vi "Magnet update rewiring.vi"(6 "output cluster":T1, 9 "Time":timestamp, 10 "Magnet in":T8, 11 "Magnet controls in":T7 {"Output\n[T]" scale=0.0..16.0; "Field\n[T]" scale=0.0..16.0; "Desired ramp\nrate [mT/s]" max=7.545; "Set Field [T]" min=0.0 max=16.0}) -> (2 "Magnet out":T8, 3 "Magnet controls out":T7 {"Output\n[T]" scale=0.0..16.0; "Field\n[T]" scale=0.0..16.0; "Desired ramp\nrate [mT/s]" max=7.545; "Set Field [T]" min=0.0 max=16.0})   [LabVIEW 2024]
uses:
  Subsystem modules/Magnet module/ctl/RampingOutput.ctl
  Datatypes/Magnet controls.ctl
  Subsystem modules/Magnet module/ctl/Overall status.ctl
  Subsystem modules/Magnet module/ctl/SetField data.ctl
  Subsystem modules/Magnet module/ctl/Magnet mode public.ctl
  Subsystem modules/Magnet module/ctl/Actual magnet state.ctl
  Subsystem modules/Magnet module/ctl/Magnet mode.ctl
  Subsystem modules/Magnet module/Magnet module.lvlib
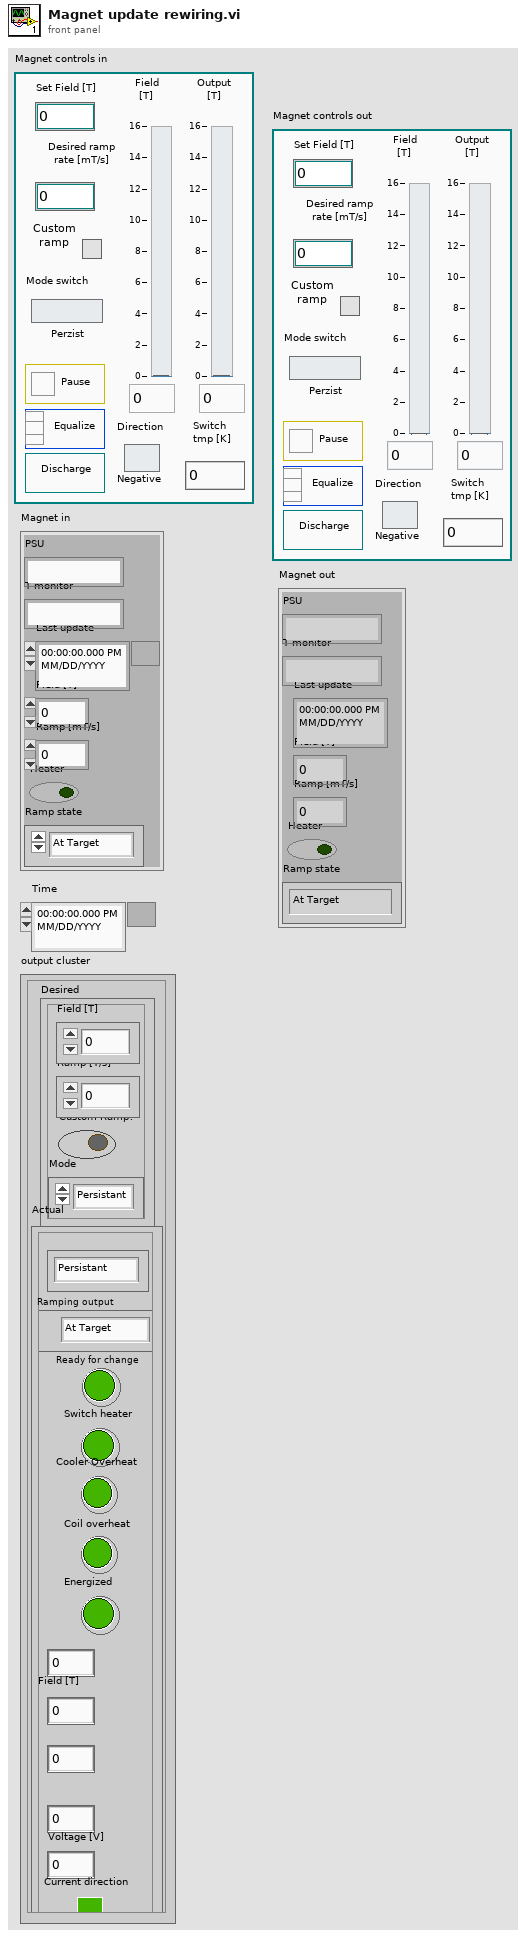
[diagram p1: front panel]
types:
  T1 = typedef "Magnet module.lvlib/Overall status.ctl" = cluster{"Desired":T2, "Actual":T4}
  T2 = typedef "Magnet module.lvlib/SetField data.ctl" = cluster{"Field [T]":dbl, "Ramp [T/s]":dbl, "Custom Ramp?":bool, "Mode":T3}
  T3 = typedef "Magnet module.lvlib/Magnet mode public.ctl" = enum16{"Persistant", "Ramping"}
  T4 = typedef "Magnet module.lvlib/Actual magnet state.ctl" = cluster{"Mode":T5, "Ramping output":T6, "Ready for change":bool, "Switch heater":bool, "Cooler Overheat":bool, "Coil overheat":bool, "Energized":bool, "Output [T]":dbl, "Field [T]":dbl, "Ramp[T/s]":dbl, "Switch\ntemperature [K]":dbl, "Voltage [V]":dbl, "Current direction":bool}
  T5 = typedef "Magnet module.lvlib/Magnet mode.ctl" = enum16{"Persistant", "Switching", "Ramping", "Quenched"}
  T6 = typedef "Magnet module.lvlib/RampingOutput.ctl" = enum16{"At Target", "Go up", "Go down"}
  T7 = typedef "Magnet controls.ctl" = cluster{"Set Field [T]":dbl, "Desired ramp\nrate [mT/s]":dbl, "Custom\nramp":bool, "Mode switch":bool, "Pause ramp":bool, "Field\n[T]":dbl, "Output\n[T]":dbl, "Equalize":bool, "Discharge":bool, "Switch \ntmp [K]":dbl, "Direction":bool}
  T8 = cluster{"PSU":string, "T monitor":string, "Last update":timestamp, "Field [T]":dbl, "Ramp [mT/s]":dbl, "Heater":bool, "Ramp state":T6}
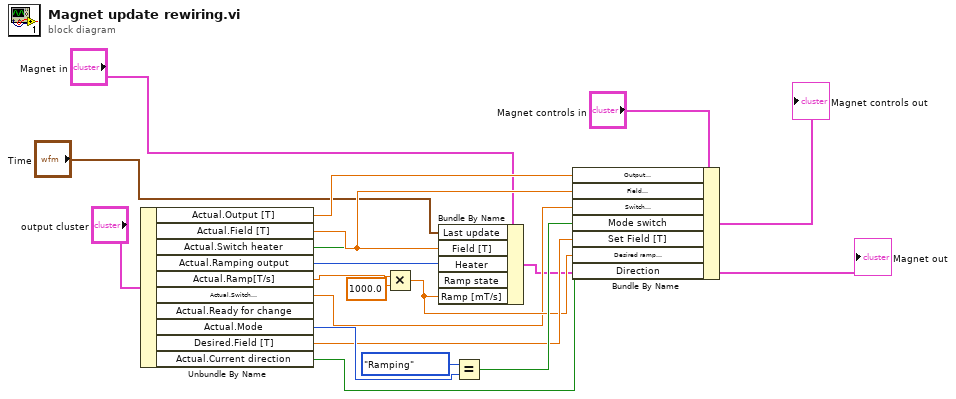
[diagram p0: block diagram]
diagram:
  n1 = Unbundle By Name("output cluster") -> ("Actual.Output [T]"=w10:dbl, "Actual.Field [T]"=w15:dbl, "Actual.Switch heater"=w3:bool, "Actual.Ramping output"=w13:T6, "Actual.Ramp[T/s]"=w11:dbl, "Actual.Switch\ntemperature [K]"=w12:dbl, "Actual.Mode"=w17:T5, "Desired.Field [T]"=w16:dbl, "Actual.Current direction"=w1:bool)  [unwired: 1 out]
  n2 = Multiply(x=w11, y=1000.0) -> (x*y=w14:dbl)
  n3 = Bundle By Name(cluster="Magnet in", "Last update"="Time", "Field [T]"=w15, "Heater"=w3, "Ramp state"=w13, "Ramp [mT/s]"=w14) -> (→"Magnet out":T8)
  n4 = Equal?(x=Magnet_mode."Ramping", y=w17) -> (x = y?=w19:bool)
  n5 = Bundle By Name(cluster="Magnet controls in", "Output\n[T]"=w10, "Field\n[T]"=w15, "Switch \ntmp [K]"=w12, "Mode switch"=w19, "Set Field [T]"=w16, "Desired ramp\nrate [mT/s]"=w14, "Direction"=w1) -> (→"Magnet controls out":T7)
